vi "count rate.vi"(8 "Acquisition time (s)":dbl, 11 "Period":dbl) -> (0 "output cluster":cluster{i32, "Period":dbl, i32[]}, 3 "counts per second":dbl(knob) scale=0.0..100.0)   [LabVIEW 2014]
uses:
  <vilib>/Platform/TimedLoop/XDataNode/timing_clust.ctl
  <vilib>/Platform/TimedLoop/XDataNode/nitl_modes.ctl
  <vilib>/Platform/TimedLoop/XDataNode/wakeup.ctl
  <vilib>/platform/TimedLoop/XDataNode/XDataNode.xnode
  <vilib>/Platform/TimedLoop/XDataNode/XDNodeRunTimeDep.lvlib
panel:
  out "Waveform Graph":cluster{i32, "Period":dbl, i32[]}(graph)
  in  "stop":bool
  # "Demo count rate VI for Physics 434"
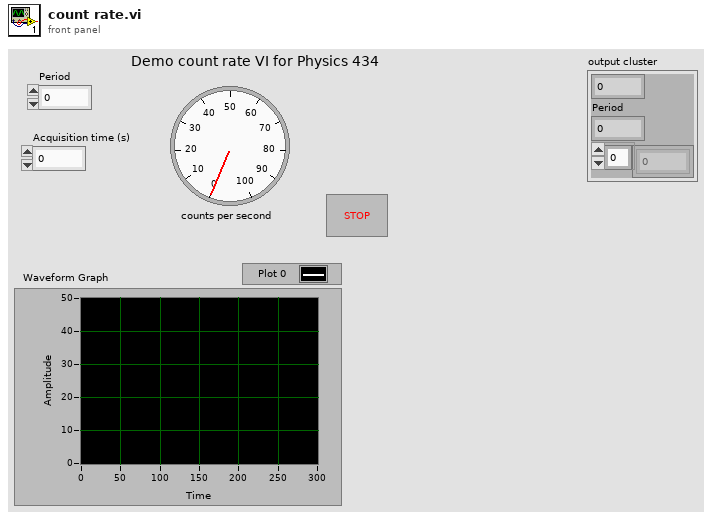
[diagram p1: front panel]
types:
  T1 = typedef "XDNodeRunTimeDep.lvlib/timing_clust.ctl" = cluster{"Expected End [f-1]":u64, "Actual End [f-1]":u64, "Finished Late? [f-1]":bool, "Expected End [i-1]":u64, "Actual End [i-1]":u64, "Finished Late? [i-1]":bool, "Expected Start [i]":u64, "Actual Start [i]":u64, "Expected Start [f]":u64, "Actual Start [f]":u64, "Source Name":string, "Structure Name":string, "Period":i64, "Deadline":i64, "Offset":i64, "Start":i64, "Priority":i32, "Timeout":i32, "Mode":T2, "Wakeup Reason":T3, "Error":errorcluster, "Source Type":string, "Secondary Source Type":string, "Global End Time":u64, "Global Start Time":u64, "Frame Duration":u64, "Iteration Duration":u64, "Assigned CPU":i32, "I/O Scan Engine Mode":u32}
  T2 = typedef "XDNodeRunTimeDep.lvlib/nitl_modes.ctl" = enum32{"No Change", "Process missed periods, maintain original phase", "Discard missed periods, maintain original phase", "Process missed periods, ignore original phase", "Discard missed periods, ignore original phase"}
  T3 = typedef "XDNodeRunTimeDep.lvlib/wakeup.ctl" = enum32{"Normal", "Aborted", "Asynchronous wakeup", "Timing source error", "Timed loop error", "Timeout"}
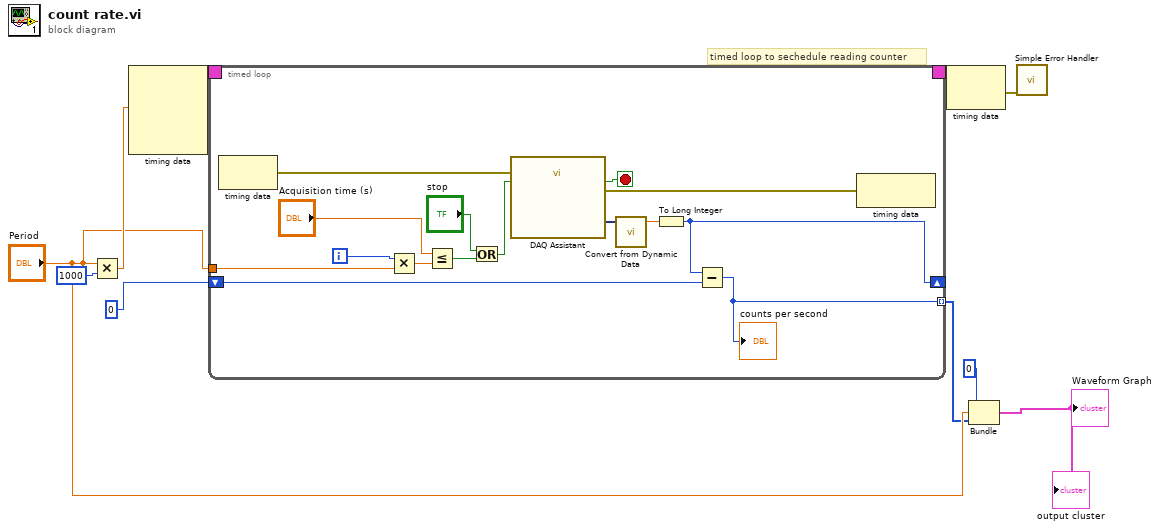
[diagram p0: block diagram]
diagram:
  # "timed loop to sechedule reading counter"
  n1 = Multiply(x="Period", y=i64 1000 ("Period")) -> (x*y=w5:dbl)
  n2 = node-c288(w5) -> (w10:T1)  [unwired: 3 in]
  n3 = timed-loop {
    timing: w10 -> [_]
    timing-out: [_] -> w9
    shift-right: [w23] -> _
    shift-left: 0 -> [w18]
    tunnel: [w19] -> w3 mode=indexing
    tunnel: "Period" -> [w17]
    i -> [w12]
    stop <- w24 stop-if-true
    n4 = node-c288() -> (w20:errorcluster)  [unwired: 1 in]
    n5 = Multiply(x=w12, y=w17) -> (x*y=w11:dbl)
    n6 = Less Or Equal?(x="Acquisition time (s)", y=w11) -> (x <= y?=w15:bool)
    n7 = Or(x="stop", y=w15) -> (x .or. y?=w13:bool)
    n8 = call "DAQ Assistant"("error in"=w20, "stop (F)"=w13) -> ("data"=w25:dynamicdata, "stopped"=w24:bool, "error out"=w21:errorcluster)  [unwired: 14 in, 1 out]
    n9 = call "Convert from Dynamic Data"("Dynamic Data Type"=w25) -> ("Scalar"=w22:dbl)  [unwired: 3 in]
    n10 = To Long Integer(number=w22) -> (32bit integer=w23:i32)
    n11 = Subtract(x=w23, y=w18) -> (x-y=w19:i32)
    "counts per second" <- w19
    n12 = node-c288(w21) -> ()  [unwired: 1 out]
  }
  n13 = node-c288(w9) -> (w7:errorcluster)
  n14 = Bundle(0, "Period"="Period", w3) -> (→"Waveform Graph" →"output cluster":cluster{i32, "Period":dbl, i32[]})  [unwired: 1 in]
  n15 = call <vilib>:"Simple Error Handler.vi"("error in (no error)"=w7) -> ()  [unwired: 4 in, 5 out]
